vi "Graphs and Fitting.vi"() -> ()   [LabVIEW 2024]
uses:
  <vilib>/Analysis/NI_AALPro.lvlib
panel:
  out "residue 2":dbl
  out "power":dbl
  out "y=x^2 Graph":T1(graph)
  in  "Array 4":dbl[](array[numeric])
  in  "Array 3":dbl[](array[numeric])
  out "residue":dbl
  out "slope":dbl
  out "y=x Graph":T2(graph)
  in  "Array 2":dbl[](array[numeric])
  in  "Array":dbl[](array[numeric])
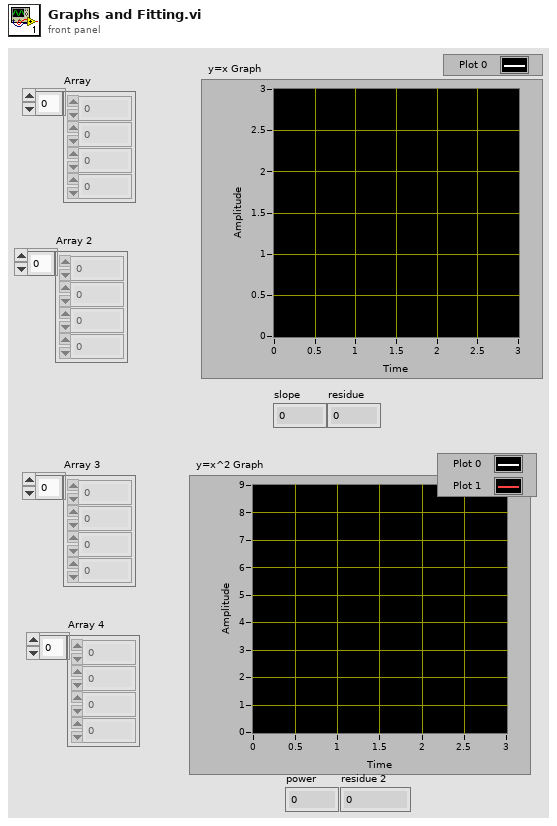
[diagram p1: front panel]
types:
  T1 = cluster{"Array 3":dbl[], "Best Linear Fit":dbl[]}[]
  T2 = cluster{"Array":dbl[], "Best Linear Fit":dbl[]}[]
  T3 = cluster{"Array 3":dbl[], "Best Power Fit":dbl[]}[]
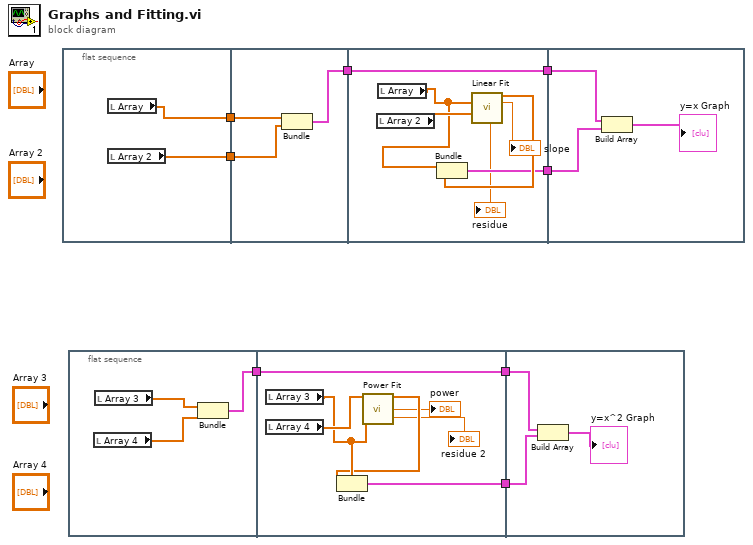
[diagram p0: block diagram]
diagram:
  n1 = flat-sequence {
    tunnel: [w10] -> w8
    tunnel: [w9] -> w7
    tunnel: w8 -> [w13]
    tunnel: w7 -> [w12]
    tunnel: [w11] -> w5
    tunnel: [w17] -> w6
    tunnel: w5 -> [w17]
    tunnel: [w16] -> w4
    tunnel: w6 -> [w23]
    tunnel: w4 -> [w22]
    frame #0 {
      n2 = local read "Array"() -> (w10:dbl[])
      n3 = local read "Array 2"() -> (w9:dbl[])
    }
    frame #1 {
      n4 = Bundle "Bundle"("Array"=w13, "Array 2"=w12) -> (w11:cluster{"Array":dbl[], "Array 2":dbl[]})  [unwired: 1 in]
    }
    frame #2 {
      n5 = local read "Array 2"() -> (w20:dbl[])
      n6 = local read "Array"() -> (w19:dbl[])
      n7 = call <vilib>:"Linear Fit.vi"("Y"=w20, "X"=w19) -> ("Best Linear Fit"=w18:dbl[], "slope"=→"slope":dbl, "residue"=→"residue":dbl)  [unwired: 9 in, 2 out]
      n8 = Bundle "Bundle"("Array"=w19, "Best Linear Fit"=w18) -> (w16:cluster{"Array":dbl[], "Best Linear Fit":dbl[]})  [unwired: 1 in]
    }
    frame #3 {
      n9 = Build Array "Build Array"(w23, w22) -> (→"y=x Graph":T2)
    }
  }
  n10 = flat-sequence {
    tunnel: [w24] -> w2
    tunnel: [w33] -> w3
    tunnel: w2 -> [w33]
    tunnel: [w29] -> w1
    tunnel: w3 -> [w36]
    tunnel: w1 -> [w35]
    frame #0 {
      n11 = local read "Array 4"() -> (w25:dbl[])
      n12 = local read "Array 3"() -> (w26:dbl[])
      n13 = Bundle("Array 3"=w26, "Array 4"=w25) -> (w24:cluster{"Array 3":dbl[], "Array 4":dbl[]})  [unwired: 1 in]
    }
    frame #1 {
      n14 = local read "Array 3"() -> (w31:dbl[])
      n15 = local read "Array 4"() -> (w32:dbl[])
      n16 = call <vilib>:"Power Fit.vi"("Y"=w32, "X"=w31) -> ("Best Power Fit"=w30:dbl[], "power"=→"power":dbl, "residue"=→"residue 2":dbl)  [unwired: 8 in, 3 out]
      n17 = Bundle("Array 3"=w31, "Best Power Fit"=w30) -> (w29:cluster{"Array 3":dbl[], "Best Power Fit":dbl[]})  [unwired: 1 in]
    }
    frame #2 {
      n18 = Build Array(w36, w35) -> (→"y=x^2 Graph":T3)
    }
  }
